vi "Create_AO_WF.vi"(8 "error in":errorcluster) -> (0 "error out":errorcluster)   [LabVIEW 2025]
panel:
  out "Illumination analog waveforms":waveform(dbl)[](graph) caption="Output Waveform"
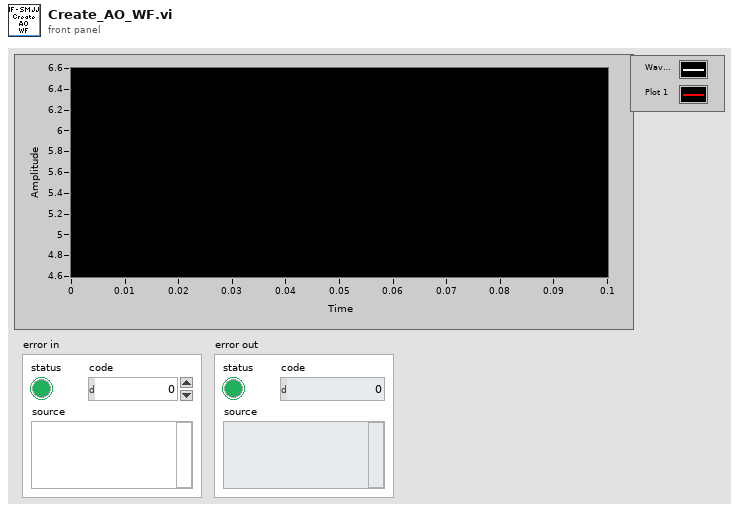
[diagram p1: front panel]
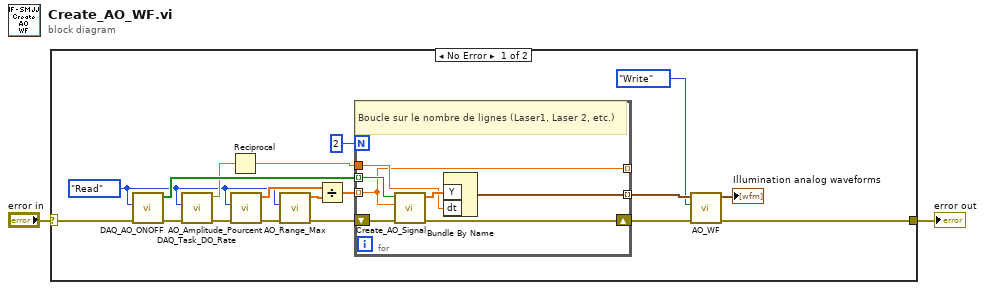
[diagram p0: block diagram]
diagram:
  n1 = case shown="No Error" "error in" {
    selector: "error in" -> [w20 w28]
    tunnel: [w18 w28] -> w1
    frame No Error {
      w5 = enum16{"Init", "Write", "Read"}."Read" ("Action")
      n2 = call "DAQ_AO_ONOFF.vi"("error in"=w20, "Action"=w5) -> ("error out"=w15:errorcluster, "AO | ON/OFF"=w17:bool[])  [unwired: 8 in]
      n3 = call "DAQ_Task_DO_Rate.vi"("error in"=w15, "Action"=w5) -> ("error out"=w11:errorcluster, "DO_Rate"=w14:dbl)  [unwired: 8 in]
      n4 = Reciprocal(x=w14) -> (1/x=w12:dbl)
      n5 = call "AO_Amplitude_Pourcent.vi"("error in"=w11, "Action"=w5) -> ("error out"=w10:errorcluster, "AO | %"=w8:dbl[])  [unwired: 8 in]
      n6 = call "AO_Range_Max.vi"("error in"=w10, "Action"=w5) -> ("error out"=w6:errorcluster, "AO | Max"=w9:dbl[])  [unwired: 8 in]
      n7 = Divide(x=w8, y=w9) -> (x/y=w7:dbl[])
      n8 = for {
        N: 2 -> [_]
        shift-right: [w22] -> w19
        shift-left: w6 -> [w27]
        tunnel: w17 -> [w26] mode=indexing
        tunnel: w12 -> [w24]
        tunnel: [w23] -> w13 mode=indexing
        tunnel: [w21] -> _ mode=indexing
        tunnel: w7 -> [w21] mode=indexing
        # "Boucle sur le nombre de lignes (Laser1, Laser 2, etc.)"
        n9 = call "Create_AO_Signal.vi"("error in"=w27, "AO Amplitude"=w21, "ON / OFF"=w26) -> ("error out"=w22:errorcluster, "WF"=w25:dbl[])  [unwired: 7 in]
        n10 = Bundle By Name("Y"=w25, "dt"=w24) -> (w23:waveform(dbl))  [unwired: 1 in]
      }
      n11 = call "AO_WF.vi"("error in"=w19, "Action"=enum16{"Init", "Write", "Read"}."Write", "AO WF"=w13) -> ("error out"=w18:errorcluster, "AO WF"=→"Illumination analog waveforms":waveform(dbl)[])  [unwired: 7 in]
    }
    frame Error {
    }
  }
  "error out" <- w1
